vi "Update Rooms List.vi"(0 "Guest Manager Model in":refnum<class "Guest Manager Model.lvclass">, 5 "All Rooms":string[](array[string]), 7 "Available Rooms":string[](array[string]), 11 "error in (no error)":errorcluster) -> (4 "Guest Manager Model out":refnum<class "Guest Manager Model.lvclass">, 15 "error out":errorcluster)   [LabVIEW 2023, in "Guest Manager Model.lvlib" / "Guest Manager Model.lvclass"]
uses:
  Guest Manager Model.lvclass
  <vilib>/ActorFramework/Actor/Actor.lvclass/Actor.ctl
  <vilib>/ActorFramework/Message Enqueuer/Message Enqueuer.lvclass/Message Enqueuer.ctl
  Guest Manager UI/Guest Manager UI Messages/Update Rooms List Msg/Update Rooms List Msg.lvclass/Update Rooms List Msg.ctl
  <vilib>/ActorFramework/Message Enqueuer/Init from Existing Queue.vi
  <vilib>/ActorFramework/Message Enqueuer/Enqueue.vi
  Guest Manager UI/Guest Manager UI Messages/Update Rooms List Msg/Update Rooms List Msg.lvclass
  <vilib>/ActorFramework/Message Priority Queue/Priority Enqueue.vi
  <vilib>/ActorFramework/Message Enqueuer/Message Enqueuer.lvclass
  Guest Manager Model.lvclass/Guest Manager Model.ctl
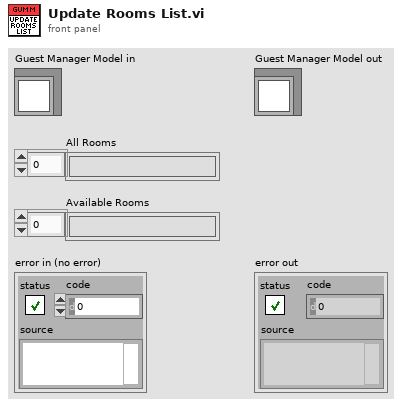
[diagram p1: front panel]
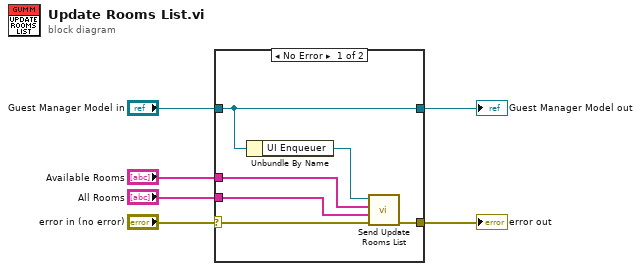
[diagram p0: block diagram]
diagram:
  n1 = case shown="No Error" "error in (no error)" {
    selector: "error in (no error)" -> [w12 w14]
    tunnel: [w11 w14] -> w5
    tunnel: [w8 w13] -> w3
    tunnel: "Guest Manager Model in" -> [w8 w13]
    tunnel: "All Rooms" -> [w9 _]
    tunnel: "Available Rooms" -> [w10 _]
    frame No Error {
      n2 = Unbundle By Name(w8) -> ("UI Enqueuer"=w7:refnum<class "Message Enqueuer.lvclass">)
      n3 = call "Send Update Rooms List.vi"("error in (no error)"=w12, "All Rooms"=w9, "Available Rooms"=w10, "Message Enqueuer"=w7) -> ("error out"=w11:errorcluster)  [unwired: 6 in, 1 out]
    }
    frame Error {
    }
  }
  "error out" <- w5
  "Guest Manager Model out" <- w3
